vi "Climber Controller.vi"(8 "error in":errorcluster) -> ()   [LabVIEW 2020]
doc: "This VI executes continuously carrying out the current operation and responding to updates or new operations. It will often contain the timing or control code that is difficult to place directly in TeleOp. This VI generally opens all sensors and motors and isolates the rest of the robot code from knowing how the operations are carried out."
uses:
  <vilib>/Rock Robotics/WPI/Framework/Completion Status.ctl
  Climber Setpoints.ctl
  Climber Operations.ctl
  Framework/Robot Global Data.vi
  <vilib>/Rock Robotics/Network Tables/NT Write Boolean.vi
panel:
  in  "Interactive Values":T1
  out "Current\nCmd":string
  in  "Buttons":cluster{"Execute Cmd":bool, "Abort Cmd":bool}
  out "Command Timing":cluster{"Start Time (ms)":u32, "Iterations":i32}
  out "Status":T3
  # "Tip: It may be helpful to observe inputs and sensor values.\nYou may also want to display tuning or debugging controls."
  # "Interactive Command: You may fill in the settings for a command\nand schedule it with the Execute button. You can observe and abort\nany command while fine tuning the code for the controller."
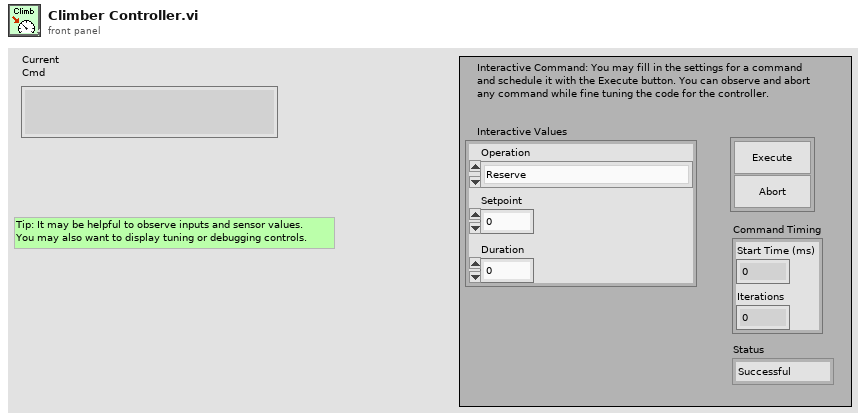
[diagram p1: front panel]
types:
  T1 = typedef "Climber Setpoints.ctl" = cluster{"Operation":T2, "Setpoint":dbl, "Duration":dbl}
  T2 = typedef "Climber Operations.ctl" = enum16{"Reserve", "Read Current", "Immediate", "climbUP", "climbDOWN"}
  T3 = typedef "Completion Status.ctl" = enum16{"Successful", "Aborted", "Incomplete"}
  T4 = typedef "WPI_MotorControlDeviceRef.ctl" = cluster{"DeviceStatus":errorcluster, "Type":T5, "PWM":cluster{"PWM Channel":T6, "DeadBand":T7}, "CAN":cluster{"Device Number":u8, "SetOutput VI Ref":variant, "GetOutput VI Ref":variant, "Enable VI Ref":variant, "Disable VI Ref":variant, "Data":variant}, "Invert":bool, "DIO PWM":cluster{"PWM \"Enable\" Channel":T6, "DIOChannel":T8, "PWM Rate":dbl}}
  T5 = typedef "WPI_MotorControlType.ctl" = enum16{"PWM", "CAN", "DIO PWM"}
  T6 = typedef "FPGA_DIOPWMChannel.ctl" = enum8{"PWM 0", "PWM 1", "PWM 2", "PWM 3", "PWM 4", "PWM 5", "PWM 6", "PWM 7", "PWM 8", "PWM 9", "PWM MXP 0", "PWM MXP 1", "PWM MXP 2", "PWM MXP 3", "PWM MXP 4", "PWM MXP 5", "PWM MXP 6", "PWM MXP 7", "PWM MXP 8", "PWM MXP 9", "Invalid"}
  T7 = typedef "WPI_PWMDeadband.ctl" = cluster{"Name":string, "maxPositivePwm":i32, "minPositivePwm":i32, "centerPwm":i32, "maxNegativePwm":i32, "minNegativePwm":i32, "angularRange":u16}
  T8 = typedef "FPGA_DIOChannel.ctl" = enum8{"DIO 0", "DIO 1", "DIO 2", "DIO 3", "DIO 4", "DIO 5", "DIO 6", "DIO 7", "DIO 8", "DIO 9", "DIO MXP 0", "DIO MXP 1", "DIO MXP 2", "DIO MXP 3", "DIO MXP 4", "DIO MXP 5", "DIO MXP 6", "DIO MXP 7", "DIO MXP 8", "DIO MXP 9", "DIO MXP 10", "DIO MXP 11", "DIO MXP 12", "DIO MXP 13", "DIO MXP 14", "DIO MXP 15", "SPI Port CS1", "SPI Port CS2", "SPI Port CS3", "SPI Port MISO", "SPI Port MOSI", "Invalid"}
  T9 = typedef "Command Status Info.ctl" = cluster{"Name":string, "Status":T3, "notifier out":T10}
  T10 = typedef "Completion Notifier.ctl" = refnum<notifier>
  T11 = cluster{"Current Command":T1, "Command Timing":cluster{"Start Time (ms)":u32, "Iterations":i32}, "Command Arguments":cluster{"Command Info":T9, "Description":string, "Default Command":T1, "queue out":refnum<queue>, "Subsystem Name":string}}
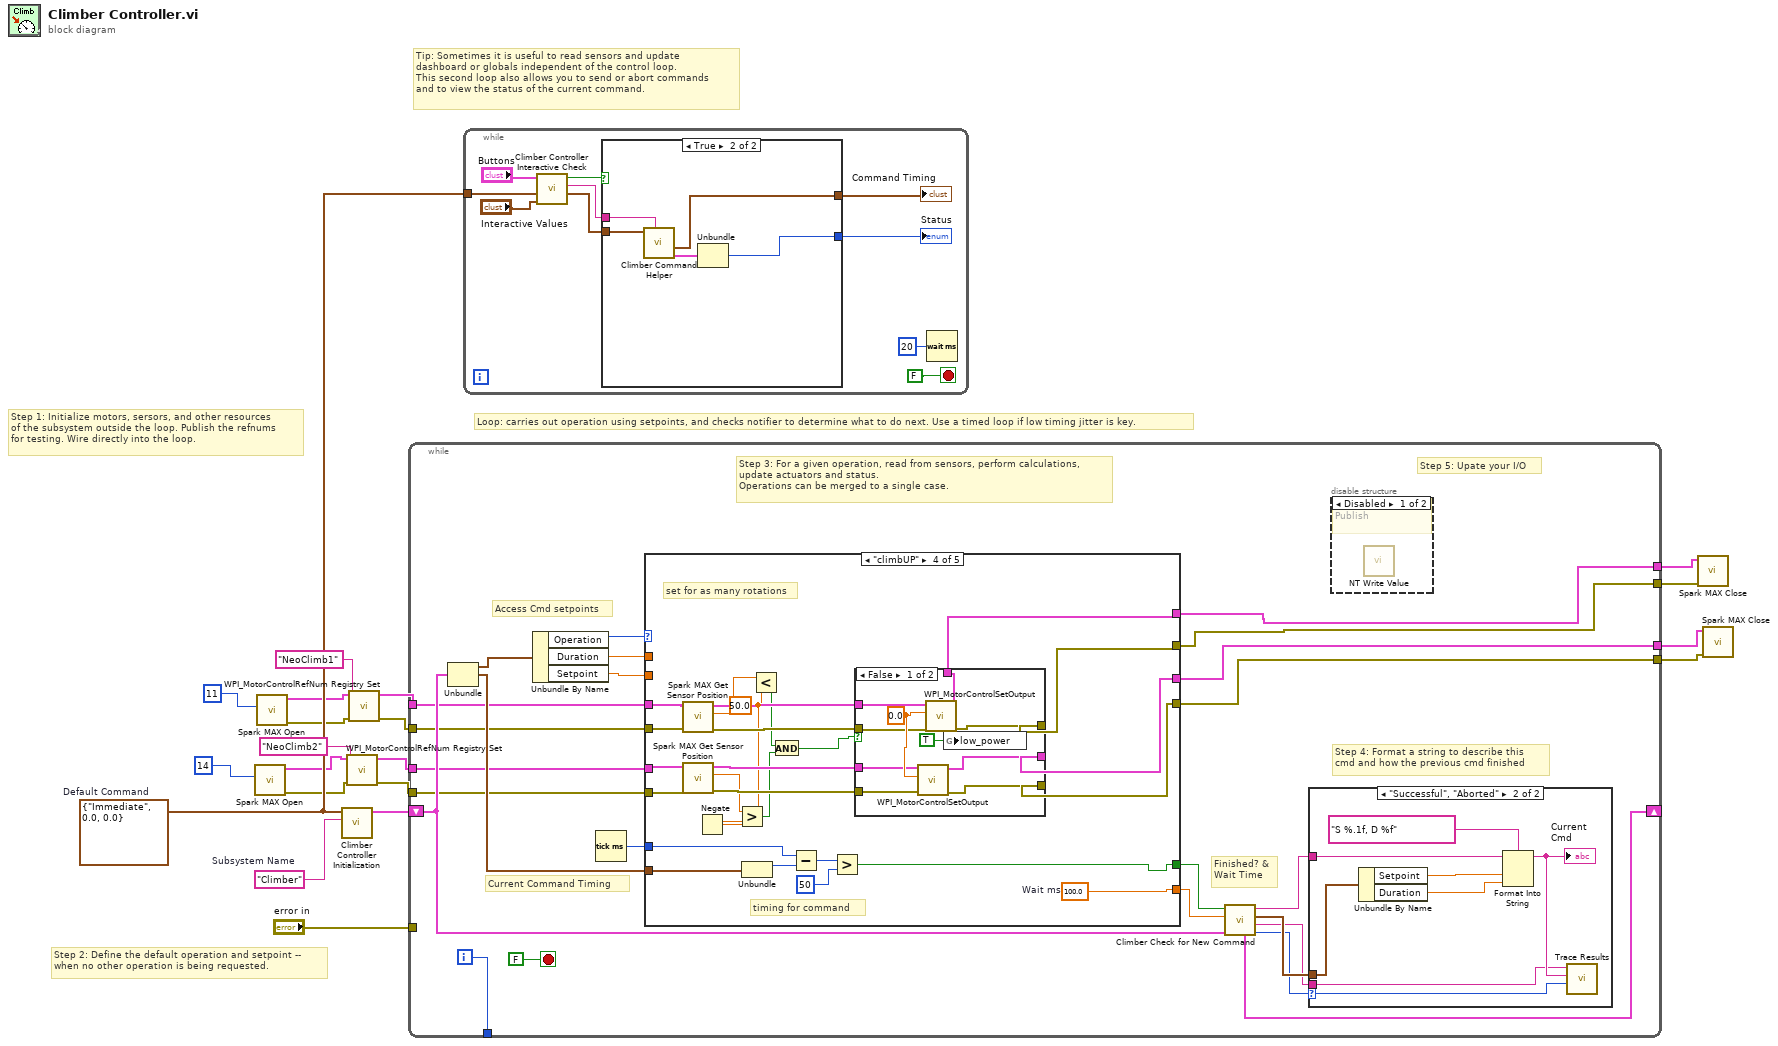
[diagram p0: block diagram]
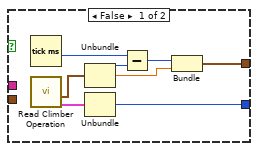
[diagram p2: hidden frame]
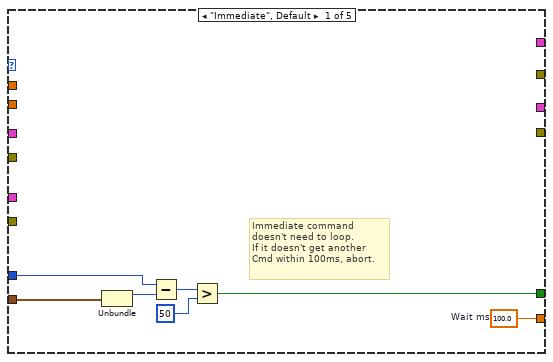
[diagram p5: hidden frame]
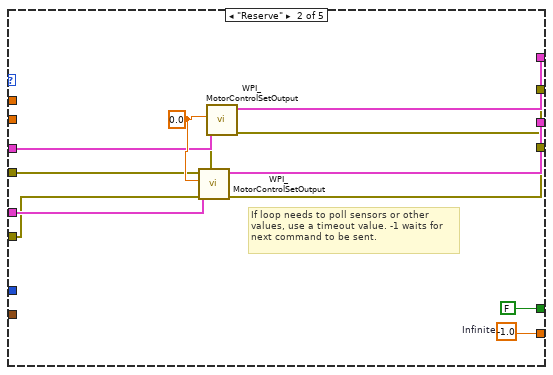
[diagram p6: hidden frame]
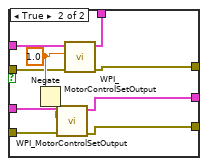
[diagram p8: hidden frame]
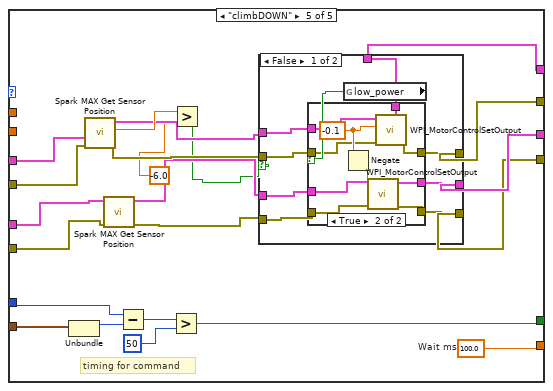
[diagram p9: hidden frame]
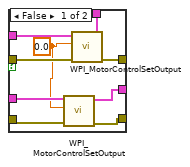
[diagram p10: hidden frame]
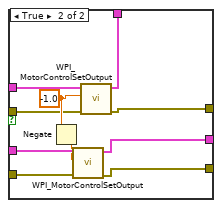
[diagram p11: hidden frame]
diagram:
  w17 = T1 {"Operation"=enum."Immediate", "Setpoint"=0.0, "Duration"=0.0}  # Default Command
  w18 = "Climber"  # Subsystem Name
  # "Tip: Sometimes it is useful to read sensors and update\ndashboard or globals independent of the control loop.\nThis second loop also allows you to send or abort commands\nand to view the status of the current command."
  # "Step 2: Define the default operation and setpoint --\nwhen no other operation is being requested."
  # "Step 1: Initialize motors, sersors, and other resources\nof the subsystem outside the loop. Publish the refnums\nfor testing. Wire directly into the loop."
  # "Loop: carries out operation using setpoints, and checks notifier to determine what to do next. Use a timed loop if low timing jitter is key."
  n1 = call <vilib>:"Spark MAX Open.vi"("Device Number"=u8 14) -> ("error out"=w4:errorcluster, "MotorControlDeviceRef"=w6:T4)  [unwired: 9 in]
  n2 = call <vilib>:"Spark MAX Open.vi"("Device Number"=u8 11) -> ("error out"=w8:errorcluster, "MotorControlDeviceRef"=w10:T4)  [unwired: 9 in]
  n3 = call "Climber Controller Initialization.vi"("Subsystem Name"=w18, "Default Command"=w17) -> ("Current Command"=w19:T11)  [unwired: 9 in]
  n4 = call <vilib>:"WPI_MotorControlRefNum Registry Set.vi"("error in (no error)"=w4, "refnum name"="NeoClimb2", "MotorControlDevRef"=w6) -> ("error out"=w3:errorcluster, "MotorControlDevRef"=w5:T4)  [unwired: 7 in]
  n5 = call <vilib>:"WPI_MotorControlRefNum Registry Set.vi"("error in (no error)"=w8, "refnum name"="NeoClimb1", "MotorControlDevRef"=w10) -> ("error out"=w7:errorcluster, "MotorControlDevRef"=w9:T4)  [unwired: 7 in]
  n6 = while {
    shift-right: [w36] -> _
    shift-left: w19 -> [w29]
    tunnel: [w43] -> _
    tunnel: "error in" -> [_]
    tunnel: w9 -> [w28]
    tunnel: w7 -> [w27]
    tunnel: w5 -> [w26]
    tunnel: w3 -> [w25]
    tunnel: [w24] -> w16
    tunnel: [w23] -> w15
    tunnel: [w22] -> w14
    tunnel: [w21] -> w13
    i -> [w43]
    stop <- FALSE stop-if-true
    # "Step 5: Upate your I/O"
    # "Step 4: Format a string to describe this\ncmd and how the previous cmd finished"
    # "Current Command Timing"
    # "Access Cmd setpoints"
    # "Finished? &\nWait Time"
    # "Step 3: For a given operation, read from sensors, perform calculations,\nupdate actuators and status.\nOperations can be merged to a single case."
    n7 = Unbundle(w29) -> ("Current Command"=w42:T1, "Command Timing"=w38:cluster{"Start Time (ms)":u32, "Iterations":i32})  [unwired: 1 out]
    n8 = Unbundle By Name(w42) -> ("Operation"=w41:T2, "Duration"=w40:dbl, "Setpoint"=w37:dbl)
    n9 = Tick Count (ms)() -> (millisecond timer value=w39:u32)
    n10 = case shown="\"climbUP\"" w41 {
      tunnel: [w59 w70 _ w90 w132] -> w34
      tunnel: [w53 FALSE ("ignore previous (F)") _ w91 w133] -> w35
      tunnel: w38 -> [w55 _ _ w93 w134]
      tunnel: w40 -> [_ _ _ _ _]
      tunnel: w39 -> [w54 _ _ w92 w135]
      tunnel: w37 -> [_ _ _ _ _]
      tunnel: w28 -> [_ w67 _ w85 w126]
      tunnel: w27 -> [_ w66 _ w83 w125]
      tunnel: w26 -> [_ w65 _ w80 w124]
      tunnel: w25 -> [_ w64 _ w79 w123]
      tunnel: [_ w61 _ w89 w131] -> w24
      tunnel: [_ w60 _ w88 w130] -> w23
      tunnel: [_ w63 _ w87 w129] -> w22
      tunnel: [_ w62 _ w86 w128] -> w21
      frame "Immediate", Default {
        w59 = 100.0  # Wait ms
        # "Immediate command\ndoesn't need to loop.\nIf it doesn't get another\nCmd within 100ms, abort."
        n11 = Unbundle(w55) -> ("Start Time (ms)"=w58:u32)  [unwired: 1 out]
        n12 = Subtract(x=w54, y=w58) -> (x-y=w57:u32)
        n13 = Greater?(x=w57, y=u8 50 ("Left Motor")) -> (0:w53:bool)
      }
      frame "Reserve" {
        w68 = 0.0 ("Output")
        w70 = -1.0  # Infinite
        # "If loop needs to poll sensors or other\nvalues, use a timeout value. -1 waits for\nnext command to be sent."
        n14 = call <vilib>:"WPI_MotorControlSetOutput.vi"("error in (no error)"=w64, "Output"=w68, "MotorControlDevRef"=w65) -> ("error out"=w62:errorcluster, "MotorControlDevRef"=w63:T4)  [unwired: 6 in, 1 out]
        n15 = call <vilib>:"WPI_MotorControlSetOutput.vi"("error in (no error)"=w66, "Output"=w68, "MotorControlDevRef"=w67) -> ("error out"=w60:errorcluster, "MotorControlDevRef"=w61:T4)  [unwired: 6 in, 1 out]
      }
      frame "Read Current" {
      }
      frame "climbUP" {
        w72 = 50.0 ("y")
        w90 = 100.0  # Wait ms
        # "set for as many rotations"
        # "timing for command"
        n16 = call <vilib>:"Spark MAX Get Sensor Position.vi"("error in (no error)"=w83, "MotorControlDevRef in"=w85) -> ("error out"=w82:errorcluster, "Sensor Position"=w77:dbl, "MotorControlDevRef out"=w84:T4)  [unwired: 6 in, 1 out]
        n17 = call <vilib>:"Spark MAX Get Sensor Position.vi"("error in (no error)"=w79, "MotorControlDevRef in"=w80) -> ("error out"=w78:errorcluster, "Sensor Position"=w76:dbl, "MotorControlDevRef out"=w81:T4)  [unwired: 6 in, 1 out]
        n18 = Negate(x=w72) -> (-x=w71:dbl)
        n19 = Greater?(x=w76, y=w71) -> (0:w74:bool)
        n20 = Unbundle(w93) -> ("Start Time (ms)"=w96:u32)  [unwired: 1 out]
        n21 = Less?(x=w77, y=w72) -> (x < y?=w75:bool)
        n22 = And(x=w75, y=w74) -> (x .and. y?=w73:bool)
        n23 = Subtract(x=w92, y=w96) -> (x-y=w95:u32)
        n24 = Greater?(x=w95, y=u8 50 ("Left Motor")) -> (0:w91:bool)
        n25 = case shown="False" w73 {
          tunnel: [w98 w115] -> w89
          tunnel: [w99 w114] -> w88
          tunnel: [w100 w113] -> w87
          tunnel: [w101 w112] -> w86
          tunnel: w84 -> [w105 w111]
          tunnel: w82 -> [w104 w110]
          tunnel: w81 -> [w103 w109]
          tunnel: w78 -> [w102 w108]
          frame False {
            w106 = 0.0 ("Output")
            n26 = call <vilib>:"WPI_MotorControlSetOutput.vi"("error in (no error)"=w102, "Output"=w106, "MotorControlDevRef"=w103) -> ("error out"=w101:errorcluster, "MotorControlDevRef"=w100:T4)  [unwired: 6 in, 1 out]
            n27 = call <vilib>:"WPI_MotorControlSetOutput.vi"("error in (no error)"=w104, "Output"=w106, "MotorControlDevRef"=w105) -> ("error out"=w99:errorcluster, "MotorControlDevRef"=w98:T4)  [unwired: 6 in, 1 out]
            n28 = global write "Robot Global Data.vi" "low_power"(TRUE ("low_power")) -> ()
          }
          frame True {
            w116 = 1.0 ("Output")
            n29 = Negate(x=w116) -> (-x=w107:dbl)
            n30 = call <vilib>:"WPI_MotorControlSetOutput.vi"("error in (no error)"=w108, "Output"=w107, "MotorControlDevRef"=w109) -> ("error out"=w112:errorcluster, "MotorControlDevRef"=w113:T4)  [unwired: 6 in, 1 out]
            n31 = call <vilib>:"WPI_MotorControlSetOutput.vi"("error in (no error)"=w110, "Output"=w116, "MotorControlDevRef"=w111) -> ("error out"=w114:errorcluster, "MotorControlDevRef"=w115:T4)  [unwired: 6 in, 1 out]
          }
        }
      }
      frame "climbDOWN" {
        w132 = 100.0  # Wait ms
        # "timing for command"
        n32 = Unbundle(w134) -> ("Start Time (ms)"=w138:u32)  [unwired: 1 out]
        n33 = call <vilib>:"Spark MAX Get Sensor Position.vi"("error in (no error)"=w125, "MotorControlDevRef in"=w126) -> ("error out"=w121:errorcluster, "Sensor Position"=w127:dbl, "MotorControlDevRef out"=w122:T4)  [unwired: 6 in, 1 out]
        n34 = call <vilib>:"Spark MAX Get Sensor Position.vi"("error in (no error)"=w123, "MotorControlDevRef in"=w124) -> ("error out"=w119:errorcluster, "MotorControlDevRef out"=w120:T4)  [unwired: 6 in, 2 out]
        n35 = Subtract(x=w135, y=w138) -> (x-y=w137:u32)
        n36 = Greater?(x=w137, y=u8 50 ("Left Motor")) -> (0:w133:bool)
        n37 = Greater?(x=w127, y=-6.0) -> (0:w117:bool)
        n38 = case shown="False" w117 {
          tunnel: [w141 w175] -> w131
          tunnel: [w140 w174] -> w130
          tunnel: [w142 w173] -> w129
          tunnel: [w143 w172] -> w128
          tunnel: w122 -> [w147 w171]
          tunnel: w121 -> [w146 w170]
          tunnel: w120 -> [w145 w169]
          tunnel: w119 -> [w144 w168]
          frame False {
            n39 = global read "Robot Global Data.vi" "low_power"() -> (w139:bool)
            n40 = case shown="True" w139 {
              tunnel: w147 -> [w156 w158]
              tunnel: w146 -> [w155 w159]
              tunnel: w145 -> [w154 w162]
              tunnel: w144 -> [w153 w163]
              tunnel: [w152 w164] -> w143
              tunnel: [w151 w165] -> w142
              tunnel: [w150 w160] -> w141
              tunnel: [w149 w161] -> w140
              frame False {
                w148 = 0.0 ("Output")
                n41 = call <vilib>:"WPI_MotorControlSetOutput.vi"("error in (no error)"=w153, "Output"=w148, "MotorControlDevRef"=w154) -> ("error out"=w152:errorcluster, "MotorControlDevRef"=w151:T4)  [unwired: 6 in, 1 out]
                n42 = call <vilib>:"WPI_MotorControlSetOutput.vi"("error in (no error)"=w155, "Output"=w148, "MotorControlDevRef"=w156) -> ("error out"=w149:errorcluster, "MotorControlDevRef"=w150:T4)  [unwired: 6 in, 1 out]
              }
              frame True {
                w166 = -0.1 ("Output")
                n43 = Negate(x=w166) -> (-x=w157:dbl)
                n44 = call <vilib>:"WPI_MotorControlSetOutput.vi"("error in (no error)"=w163, "Output"=w157, "MotorControlDevRef"=w162) -> ("error out"=w164:errorcluster, "MotorControlDevRef"=w165:T4)  [unwired: 6 in, 1 out]
                n45 = call <vilib>:"WPI_MotorControlSetOutput.vi"("error in (no error)"=w159, "Output"=w166, "MotorControlDevRef"=w158) -> ("error out"=w161:errorcluster, "MotorControlDevRef"=w160:T4)  [unwired: 6 in, 1 out]
              }
            }
          }
          frame True {
            w176 = -1.0 ("Output")
            n46 = Negate(x=w176) -> (-x=w167:dbl)
            n47 = call <vilib>:"WPI_MotorControlSetOutput.vi"("error in (no error)"=w168, "Output"=w167, "MotorControlDevRef"=w169) -> ("error out"=w172:errorcluster, "MotorControlDevRef"=w173:T4)  [unwired: 6 in, 1 out]
            n48 = call <vilib>:"WPI_MotorControlSetOutput.vi"("error in (no error)"=w170, "Output"=w176, "MotorControlDevRef"=w171) -> ("error out"=w174:errorcluster, "MotorControlDevRef"=w175:T4)  [unwired: 6 in, 1 out]
          }
        }
      }
    }
    n49 = call "Climber Check for New Command.vi"("Current Command"=w29, "Wait time (ms)"=w34, "Finished?"=w35) -> ("Completion"=w30:T3, "Subsystem Name"=w31:string, "Current Command"=w32:T1, "Initial Trace String"=w33:string, "NextCommand"=w36:T11)  [unwired: 4 in]
    n50 = case shown="\"Successful\", \"Aborted\"" w30 {
      selector: w30 -> [_ w52]
      tunnel: w33 -> [_ w48]
      tunnel: w32 -> [_ w49]
      tunnel: w31 -> [_ w45]
      frame "Incomplete", Default {
        # "Continuing current command"
      }
      frame "Successful", "Aborted" {
        # "Report and setup for next command"
        n51 = Unbundle By Name(w49) -> ("Setpoint"=w51:dbl, "Duration"=w46:dbl)
        n52 = Format Into String(format string="S %.1f, D %f", initial string=w48, w51, w46) -> (resulting string=w47:string)  [unwired: 1 in, 1 out]
        "Current\nCmd" <- w47
        n53 = call <vilib>:"Trace Results.vi"("Status of previous command"=w52, "Description"=w47, "Subsystem"=w45) -> ()  [unwired: 9 in]
      }
    }
    n54 = disable-structure shown="Disabled" {
      frame Disabled {
        # "Publish"
        n55 = call-poly <vilib>:"NT Write Value.vi"() -> ()  [unwired: 11 in, 1 out]
      }
      frame Enabled {
      }
    }
  }
  n56 = while {
    tunnel: w17 -> [w183]
    stop <- FALSE stop-if-true
    n57 = call "Climber Controller Interactive Check.vi"("Interactive Command in"="Interactive Values", "Default Command"=w183, "Buttons"="Buttons") -> ("Interactive Command out"=w180:T1, "Trace String"=w181:string, "Schedule"=w182:bool)  [unwired: 6 in]
    n58 = case shown="True" w182 {
      tunnel: [w194 w199] -> w179
      tunnel: w180 -> [_ w197]
      tunnel: [w190 w195] -> w178
      tunnel: w181 -> [_ w198]
      frame False {
        n59 = Tick Count (ms)() -> (millisecond timer value=w189:u32)
        n60 = call "Read Climber Operation.vi"() -> ("Command Info"=w187:T9, "SubSystem Data"=w188:T1)  [unwired: 9 in, 1 out]
        n61 = Unbundle(w188) -> ("Operation"=w193:T2, "Setpoint"=w191:dbl)  [unwired: 1 out]
        n62 = Unbundle(w187) -> ("Status"=w194:T3)  [unwired: 2 out]
        n63 = Subtract(x=w189, y=w193) -> (x-y=w192:u32)
        n64 = Bundle(w192, "Setpoint"=w191) -> (w190:cluster{u32, "Setpoint":dbl})  [unwired: 1 in]
      }
      frame True {
        n65 = call "Climber Command Helper.vi"("Description"=w198, "SubSystem Data"=w197) -> ("Command Info Out"=w196:T9, "Command Timing"=w195:cluster{"Start Time (ms)":u32, "Iterations":i32})  [unwired: 7 in, 1 out]
        n66 = Unbundle(w196) -> ("Status"=w199:T3)  [unwired: 2 out]
      }
    }
    "Status" <- w179
    "Command Timing" <- w178
    n67 = Wait (ms)(milliseconds to wait=u32 20) -> ()  [unwired: 1 out]
  }
  n68 = call <vilib>:"Spark MAX Close.vi"("error in"=w15, "MotorControlDeviceRef"=w16) -> ()  [unwired: 9 in, 1 out]
  n69 = call <vilib>:"Spark MAX Close.vi"("error in"=w13, "MotorControlDeviceRef"=w14) -> ()  [unwired: 9 in, 1 out]
